vi "CFG Find Delimiter.vi"(0 "Value":string, 7 "Dimensions":i32, 11 "Error In (no error)":errorcluster) -> (8 "Delimiter (s)":string, 15 "Error Out":errorcluster)   [LabVIEW 2012]
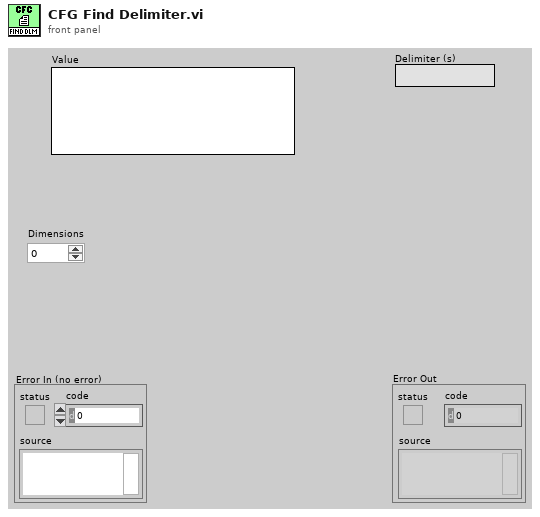
[diagram p1: front panel]
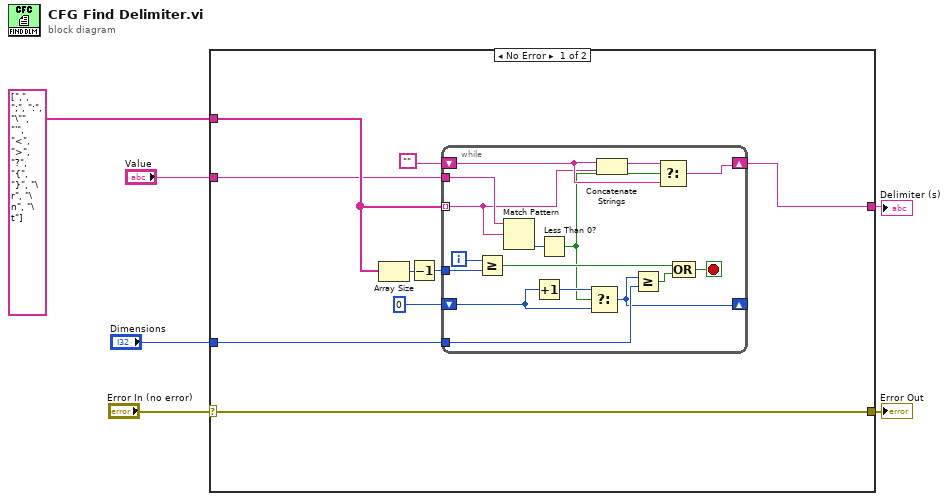
[diagram p0: block diagram]
diagram:
  n1 = case shown="No Error" "Error In (no error)" {
    selector: "Error In (no error)" -> [w12 w32]
    tunnel: [w12 w32] -> w6
    tunnel: [w8 _] -> w5
    tunnel: string[] [",", ";", ":", "\"", "'", "<", ">", "?", "{", "}", "\r", "\n", "\t"] -> [w15 _]
    tunnel: "Value" -> [w7 _]
    tunnel: "Dimensions" -> [w10 _]
    frame No Error {
      n2 = Array Size(array=w15) -> (size(s)=w14:i32)
      n3 = Decrement(x=w14) -> (x-1=w13:i32)
      n4 = while {
        tunnel: w13 -> [w29]
        tunnel: w15 -> [w19] mode=indexing
        tunnel: w7 -> [w31]
        shift-right: [w23] -> _
        shift-left: 0 -> [w22]
        tunnel: w10 -> [w24]
        shift-right: [w16] -> w8
        shift-left: "" -> [w20]
        i -> [w30]
        stop <- w28 stop-if-true
        n5 = Greater Or Equal?(x=w30, y=w29) -> (x >= y?=w27:bool)
        n6 = Match Pattern(string=w31, regular expression=w19) -> (offset past match=w26:i32)  [unwired: 4 out]
        n7 = Increment(x=w22) -> (x+1=w25:i32)
        n8 = Less Than 0?(x=w26) -> (x < 0?=w17:bool)
        n9 = Select(t=w25, s=w17, f=w22) -> (s? t:f=w23:i32)
        n10 = Concatenate Strings(w20, w19) -> (w18:string)
        n11 = Greater Or Equal?(x=w23, y=w24) -> (x >= y?=w21:bool)
        n12 = Select(t=w18, s=w17, f=w20) -> (s? t:f=w16:string)
        n13 = Compound Arithmetic op=OR(w27, w21) -> (w28:bool)
      }
    }
    frame Error {
    }
  }
  "Error Out" <- w6
  "Delimiter (s)" <- w5
